vi "Ctor.vi"(8 "error in (no error)":errorcluster) -> (0 "error out":errorcluster, 3 "Manager out":refnum<class "Manager.lvclass">)   [LabVIEW 2020, in "OOPanel.lvlib" / "Manager.lvclass"]
uses:
  Manager.lvclass
  Ref Data.ctl
  SubPanel Map.ctl
  Panel/Panel.lvclass
  Manager.lvclass/Manager.ctl
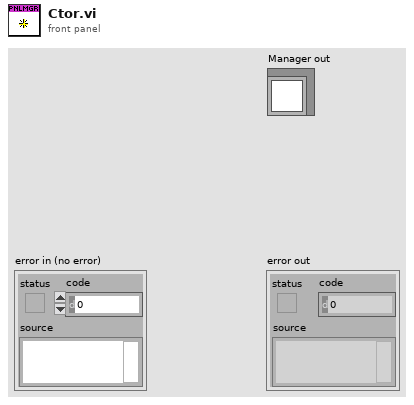
[diagram p1: front panel]
types:
  T1 = typedef "OOPanel.lvlib/Manager.lvclass/Ref Data.ctl" = cluster{"SubPanel Map":T2, "Panels":refnum<class "Panel.lvclass">[]}
  T2 = typedef "OOPanel.lvlib/Manager.lvclass/SubPanel Map.ctl" = cluster{"SubPanels":refnum<vi>[], "Panels":refnum<class "Panel.lvclass">[]}
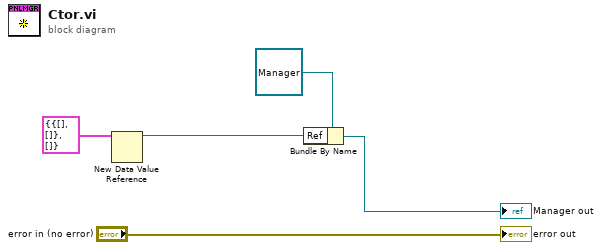
[diagram p0: block diagram]
diagram:
  n1 = New Data Value Reference(data value=T1 {"SubPanel Map"={"SubPanels"=[], "Panels"=[]}, "Panels"=[]} ("Ref Data")) -> (data value reference=w1:refnum<data-value>)  [unwired: 1 in, 1 out]
  n2 = Bundle By Name(cluster=refnum<class "Manager.lvclass"> refnum ("Manager in"), "Ref"=w1) -> (→"Manager out":refnum<class "Manager.lvclass">)
  "error out" <- "error in (no error)"
